vi "Read SPI.vi"(4 "CS Active Low (T)":bool=TRUE, 5 "CS Pin (None)":i32=-1, 7 "Bus":u8, 8 "error in (no error)":errorcluster, 9 "Len":u8, 11 "VISA resource name in":refnum<visa-resource-name>) -> (0 "error out":errorcluster, 1 "Data":string, 3 "VISA resource name":refnum<visa-resource-name>)   [LabVIEW 2024, in "CTIPicoVISA.lvlib"]
uses:
  CTIPicoVISA.lvlib
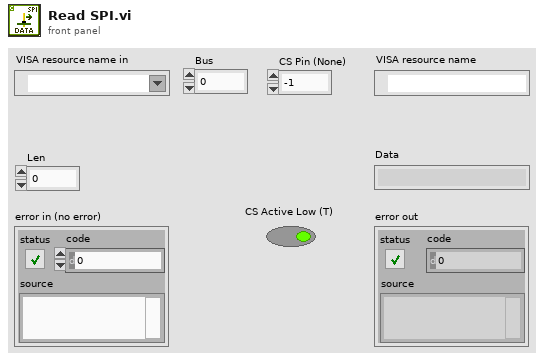
[diagram p1: front panel]
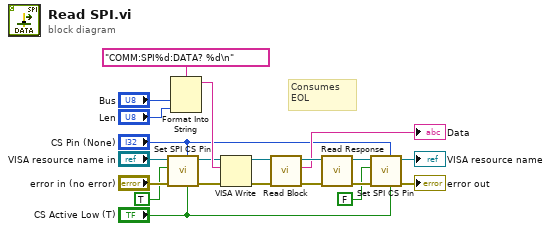
[diagram p0: block diagram]
diagram:
  # "Consumes EOL"
  n1 = call "Set SPI CS Pin.vi"("CS Active Low (T)"="CS Active Low (T)", "CS GPIO"="CS Pin (None)", "error in (no error)"="error in (no error)", "CS Active"=TRUE, "VISA resource name in"="VISA resource name in") -> ("error out"=w10:errorcluster, "VISA resource name"=w9:refnum<visa-resource-name>)  [unwired: 5 in]
  n2 = Format Into String(format string="COMM:SPI%d:DATA? %d\n", "Bus", "Len") -> (resulting string=w13:string)  [unwired: 2 in, 1 out]
  n3 = VISA Write(VISA resource name=w9, write buffer=w13, error in (no error)=w10) -> (VISA resource name out=w18:refnum<visa-resource-name>, error out=w19:errorcluster)  [unwired: 1 out]
  n4 = call "Read Block.vi"("error in (no error)"=w19, "VISA resource name in"=w18) -> ("error out"=w17:errorcluster, "Data"=→"Data":string, "VISA resource name"=w16:refnum<visa-resource-name>)  [unwired: 7 in]
  n5 = call "Read Response.vi"("error in (no error)"=w17, "VISA resource name"=w16) -> ("error out"=w7:errorcluster, "VISA resource name Out"=w6:refnum<visa-resource-name>)  [unwired: 6 in, 2 out]
  n6 = call "Set SPI CS Pin.vi"("CS Active Low (T)"="CS Active Low (T)", "CS GPIO"="CS Pin (None)", "error in (no error)"=w7, "CS Active"=FALSE, "VISA resource name in"=w6) -> ("error out"=→"error out":errorcluster, "VISA resource name"=→"VISA resource name":refnum<visa-resource-name>)  [unwired: 5 in]
